vi "clFileReader_writeToFile.vi"(8 "filename (use dialog)":path, 11 "clFileReader.lvclass IN":refnum<class "clFileReader.lvclass">) -> (0 "no Error":bool)   [LabVIEW 2021, in "vi_lib.lvlib" / "clFileReader.lvclass"]
uses:
  clFileReader.lvclass
  clFileReader.lvclass/clFileReader.ctl
  clFile/clFile.lvclass
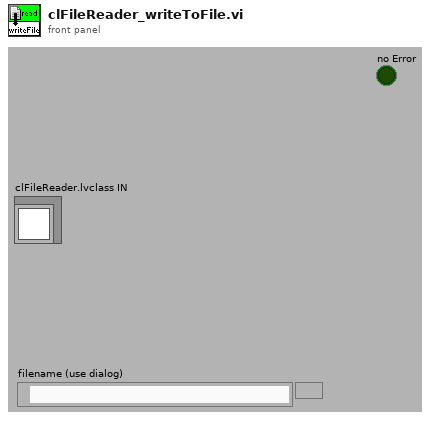
[diagram p1: front panel]
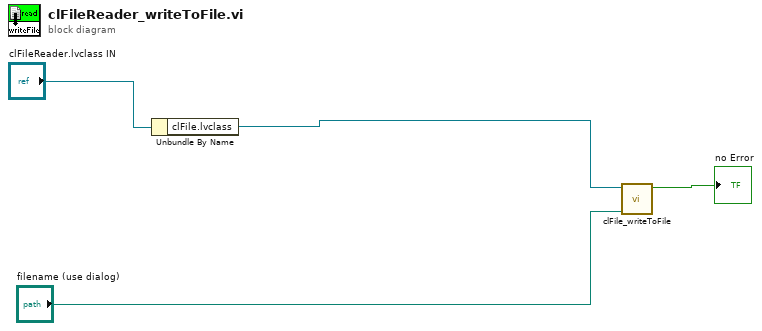
[diagram p0: block diagram]
diagram:
  n1 = Unbundle By Name("clFileReader.lvclass IN") -> ("clFile.lvclass"=w3:refnum<class "clFile.lvclass">)
  n2 = call "clFile_writeToFile.vi"("filename (use dialog)"="filename (use dialog)", "clFile.lvclass"=w3) -> ("no Error"=→"no Error":bool)  [unwired: 9 out]
